vi "Save txt.vi"(8 "error in (no error)":errorcluster, 10 "Save?":bool, 11 "Counter in":refnum<class "Counter.lvclass">) -> (0 "error out":errorcluster, 3 "Counter out":refnum<class "Counter.lvclass">)   [LabVIEW 2019, in "Counter.lvlib" / "Counter.lvclass"]
uses:
  Counter.lvclass
  Counter.lvclass/Counter.ctl
  Save txt Messages/Save Msg/Save Msg.lvclass/Save Msg.ctl
  <vilib>/ActorFramework/Message Enqueuer/Message Enqueuer.lvclass/Message Enqueuer.ctl
  Save tdms Messages/Save Msg/Save Msg.lvclass/Save Msg.ctl
  <vilib>/ActorFramework/Message Enqueuer/Enqueue.vi
  Save txt Messages/Save Msg/Save Msg.lvclass
  C:/Program Files/National Instruments/LabVIEW 2019/vi.lib/ActorFramework/Message/Message.lvclass
  Save tdms Messages/Save Msg/Save Msg.lvclass
  <vilib>/ActorFramework/Message Priority Queue/Priority Enqueue.vi
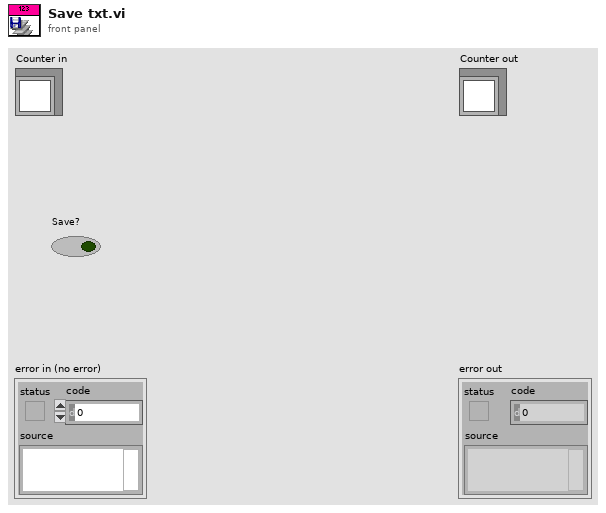
[diagram p1: front panel]
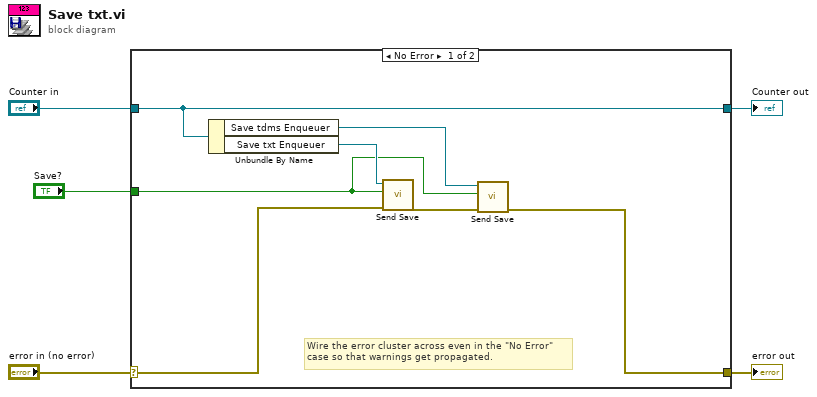
[diagram p0: block diagram]
diagram:
  n1 = case shown="No Error" "error in (no error)" {
    selector: "error in (no error)" -> [w10 w14]
    tunnel: [w7 w14] -> w4
    tunnel: [w12 w13] -> w2
    tunnel: "Counter in" -> [w12 w13]
    tunnel: "Save?" -> [w6 _]
    frame No Error {
      # "Wire the error cluster across even in the \"No Error\"\ncase so that warnings get propagated."
      n2 = Unbundle By Name(w12) -> ("Save tdms Enqueuer"=w8:refnum<class "Message Enqueuer.lvclass">, "Save txt Enqueuer"=w11:refnum<class "Message Enqueuer.lvclass">)
      n3 = call "Send Save.vi"("error in (no error)"=w10, "Save?"=w6, "Message Enqueuer"=w11) -> ("error out"=w9:errorcluster)  [unwired: 7 in, 1 out]
      n4 = call "Send Save.vi"("error in (no error)"=w9, "Save?"=w6, "Message Enqueuer"=w8) -> ("error out"=w7:errorcluster)  [unwired: 7 in, 1 out]
    }
    frame Error {
    }
  }
  "error out" <- w4
  "Counter out" <- w2
